vi "Interpret.vi"(8 "error in (no error)":errorcluster, 10 "Interpreted In":refnum<class "Interpreted.lvclass">, 11 "Interpreter in":refnum<class "Interpreter.lvclass">) -> (0 "error out":errorcluster, 2 "Interpreted Out":refnum<class "Interpreted.lvclass">, 3 "Interpreter out":refnum<class "Interpreter.lvclass">)   [LabVIEW 2022 SP3, in "Interpreter.lvclass"]
uses:
  Interpreter.lvclass
  Interpreted/Interpreted.lvclass
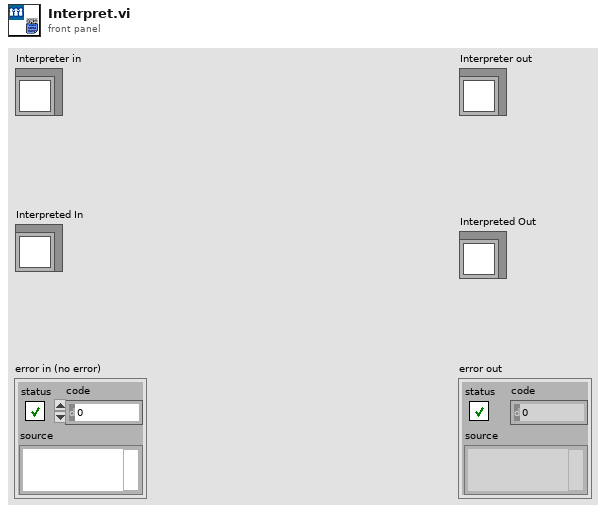
[diagram p1: front panel]
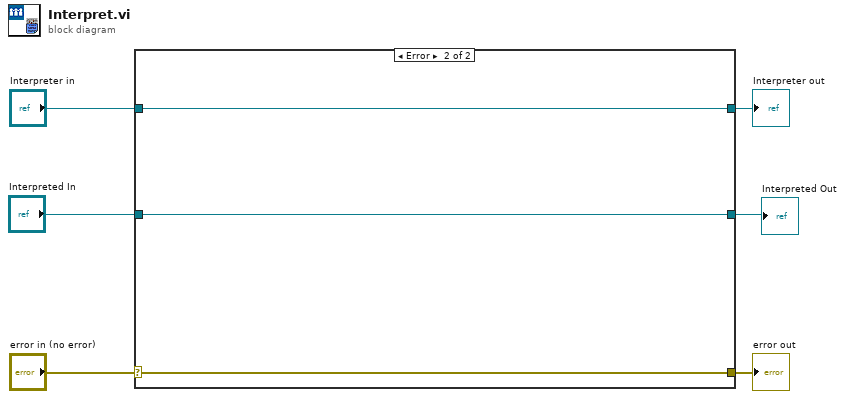
[diagram p0: block diagram]
diagram:
  n1 = case shown="Error" "error in (no error)" {
    selector: "error in (no error)" -> [w8 w12]
    tunnel: [w8 w12] -> w5
    tunnel: [w9 w11] -> w3
    tunnel: "Interpreter in" -> [w9 w11]
    tunnel: [w7 w10] -> w2
    tunnel: "Interpreted In" -> [w7 w10]
    frame No Error {
      # "Wire the error cluster across even in the \"No Error\"\ncase so that warnings get propagated."
    }
    frame Error {
    }
  }
  "error out" <- w5
  "Interpreter out" <- w3
  "Interpreted Out" <- w2
